vi "Customize Meter.vi"() -> ()   [LabVIEW 2019, in "Instrument.OxfordVRM UI.lvclass"]
uses:
  Instrument.OxfordVRM UI.lvclass
  <vilib>/Utility/miscctls.llb/LVBoundsTypeDef.ctl
panel:
  out "Magnet Field (T) 2":dbl(knob) caption="Voltage (V)" scale=-50.0..50.0
  out "Meter 2":dbl(knob) scale=-50.0..50.0
  in  "Housing Size":T1
  in  "Scale.Interpolate Color":bool
  in  "Color 3":u32(colorbox)=16776960
  in  "Color 2":u32(colorbox)=16860
  in  "Color 1":u32(colorbox)=16744448
  in  "Limit 4":dbl=50.0
  in  "Limit 3":dbl=30.0
  in  "Limit 2":dbl=6.0
  in  "Limit 1":dbl=-6.0
  out "Meter":dbl(knob)=21.586596923816817 scale=-50.0..50.0
  out "Meter Scale.Marker Values":cluster{"Limit":dbl, "Color":u32}[](array[cluster])=[{"Limit"=-6.0, "Color"=16744448}, {"Limit"=6.0, "Color"=16860}, {"Limit"=30.0, "Color"=16776960}, {"Limit"=50.0, "Color"=16776960}]
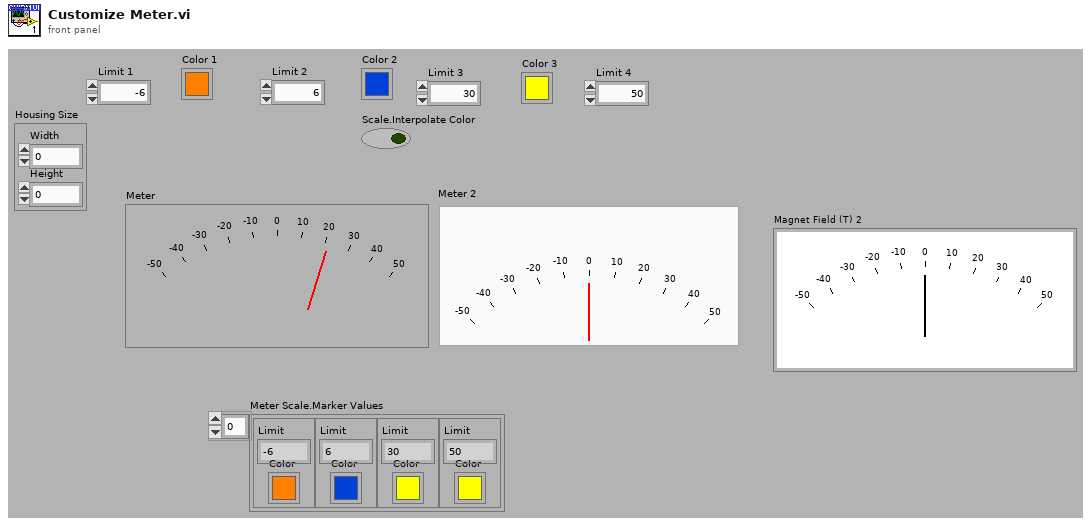
[diagram p1: front panel]
types:
  T1 = typedef "LVBoundsTypeDef.ctl" = cluster{"Width":u32, "Height":u32}
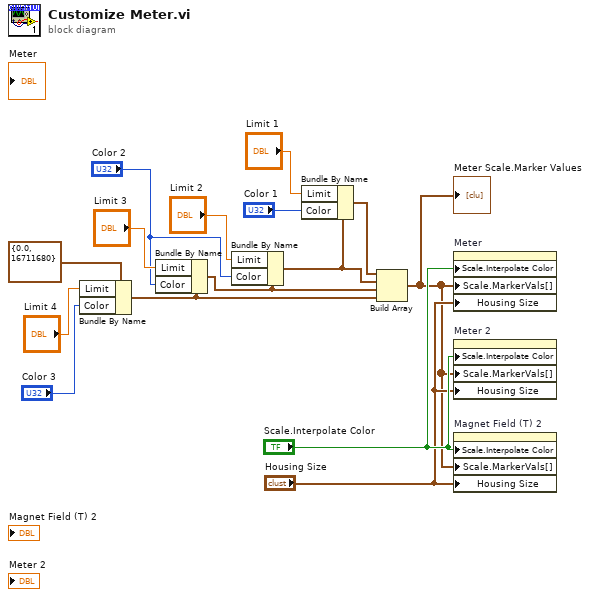
[diagram p0: block diagram]
diagram:
  n1 = Bundle By Name(cluster=cluster{"Limit":dbl, "Color":u32} {"Limit"=0.0, "Color"=16711680}, "Limit"="Limit 4", "Color"="Color 3") -> (w10:cluster{"Limit":dbl, "Color":u32})
  n2 = Bundle By Name(cluster=w10, "Limit"="Limit 3", "Color"="Color 2") -> (w11:cluster{"Limit":dbl, "Color":u32})
  n3 = Bundle By Name(cluster=w11, "Limit"="Limit 2", "Color"="Color 2") -> (w12:cluster{"Limit":dbl, "Color":u32})
  n4 = Bundle By Name(cluster=w12, "Limit"="Limit 1", "Color"="Color 1") -> (w13:cluster{"Limit":dbl, "Color":u32})
  n5 = Build Array(w13, w12, w11, w10) -> (w1:cluster{"Limit":dbl, "Color":u32}[])
  "Meter Scale.Marker Values" <- w1
  n6 = property on="Meter" class="Knob (strict)"("Scale.Interpolate Color"="Scale.Interpolate Color", "Scale.MarkerVals[]"=w1, "Housing Size"="Housing Size") -> ()  [unwired: 2 in, 2 out]
  n7 = property on="Meter 2" class="Knob (strict)"("Scale.Interpolate Color"="Scale.Interpolate Color", "Scale.MarkerVals[]"=w1, "Housing Size"="Housing Size") -> ()  [unwired: 2 in, 2 out]
  n8 = property on="Magnet Field (T) 2" class="Knob (strict)"("Scale.Interpolate Color"="Scale.Interpolate Color", "Scale.MarkerVals[]"=w1, "Housing Size"="Housing Size") -> ()  [unwired: 2 in, 2 out]
